vi "subImage.vi"() -> ()   [LabVIEW 2018]
doc: "Sublmage: This example is an example of a sub image, which can be a partial image extracted or captured from the original image."
uses:
  vi.lib/VIRobotics/opencv_yiku/ctls/Point.ctl
  vi.lib/VIRobotics/opencv_yiku/ctls/Rect.ctl
  vi.lib/VIRobotics/opencv_yiku/ctls/ColorConversionCodes.ctl
  vi.lib/VIRobotics/opencv_yiku/Mat/Mat_8U/Mat_8U.lvclass
  D:/Program Files/company/National Instruments/LabVIEW 2018/vi.lib/addons/VIRobotics/opencv_yiku/Mat/Mat/Mat.lvclass
  vi.lib/VIRobotics/opencv_yiku/Mat/Create_Mat_8U.vi
  vi.lib/VIRobotics/opencv_yiku/Cap/Cap.lvclass
  vi.lib/VIRobotics/opencv_yiku/opencv_yiku.lvlib
  vi.lib/VIRobotics/opencv_yiku/Mat/Mat/Mat.lvclass
panel:
  out "sub picture":picture
  out "replace picture":picture
  in  "sub Rect":T1={"x"=100, "y"=100, "width"=200, "height"=100}
  in  "replace start Point":T2={"x"=50, "y"=50}
  out "src picture":picture
  in  "stop":bool
  # "Overview: Demonstrates how to get a subimage and replaceSubImage\nRequirements: Windows.\nInstructions: \n1.Run the VI.\n2.Please note that the selected sub area you set must not exceed the boundaries of the image itself. The area you replace must also not exceed the boundaries of the image itself.\n3.Make sure your computer has a camera."
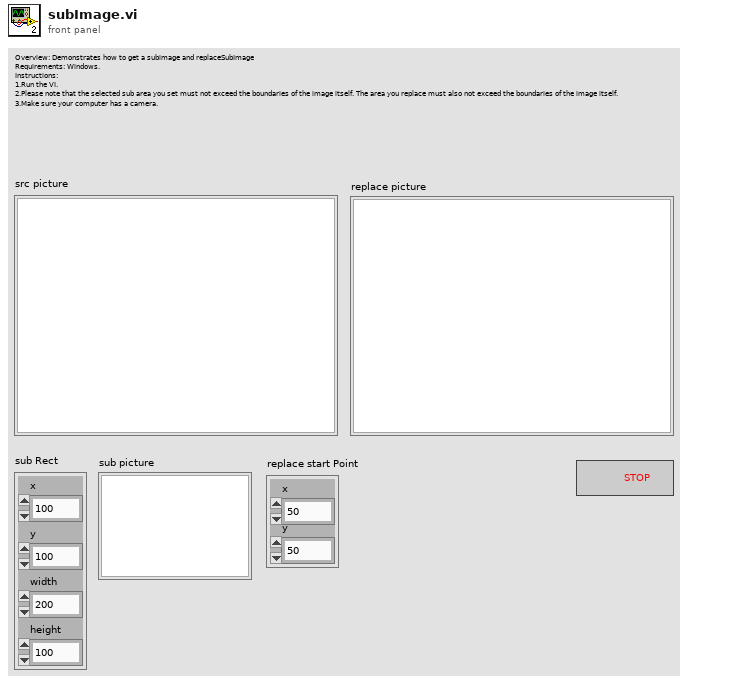
[diagram p1: front panel]
types:
  T1 = typedef "opencv_yiku.lvlib/Rect.ctl" = cluster{"x":i32, "y":i32, "width":i32, "height":i32}
  T2 = typedef "opencv_yiku.lvlib/Point.ctl" = cluster{"x":i32, "y":i32}
  T3 = typedef "opencv_yiku.lvlib/ColorConversionCodes.ctl" = enum32{"COLOR_BGR2BGRA", "COLOR_BGRA2BGR", "COLOR_BGR2RGBA", "COLOR_RGBA2BGR", "COLOR_BGR2RGB", "COLOR_BGRA2RGBA", "COLOR_BGR2GRAY", "COLOR_RGB2GRAY", "COLOR_GRAY2BGR", "COLOR_GRAY2BGRA", "COLOR_BGRA2GRAY", "COLOR_RGBA2GRAY", "COLOR_BGR2BGR565", "COLOR_RGB2BGR565", "COLOR_BGR5652BGR", "COLOR_BGR5652RGB", "COLOR_BGRA2BGR565", "COLOR_RGBA2BGR565", "COLOR_BGR5652BGRA", "COLOR_BGR5652RGBA", "COLOR_GRAY2BGR565", "COLOR_BGR5652GRAY", "COLOR_BGR2BGR555", "COLOR_RGB2BGR555", "COLOR_BGR5552BGR", "COLOR_BGR5552RGB", "COLOR_BGRA2BGR555", "COLOR_RGBA2BGR555", "COLOR_BGR5552BGRA", "COLOR_BGR5552RGBA", "COLOR_GRAY2BGR555", "COLOR_BGR5552GRAY", "COLOR_BGR2XYZ", "COLOR_RGB2XYZ", "COLOR_XYZ2BGR", "COLOR_XYZ2RGB", "COLOR_BGR2YCrCb", "COLOR_RGB2YCrCb", "COLOR_YCrCb2BGR", "COLOR_YCrCb2RGB", "COLOR_BGR2HSV", "COLOR_RGB2HSV", "42", "43", "COLOR_BGR2Lab", "COLOR_RGB2Lab"}
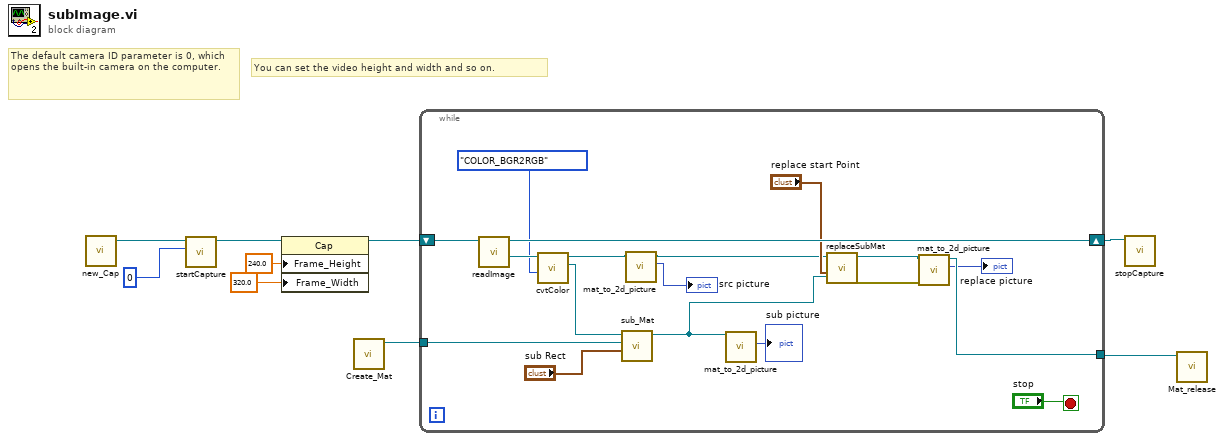
[diagram p0: block diagram]
diagram:
  # "You can set the video height and width and so on."
  # "The default camera ID parameter is 0, which opens the built-in camera on the computer."
  n1 = call "new_Cap.vi"() -> ("Cap out"=w9:refnum<class "Cap.lvclass">)  [unwired: 10 in, 1 out]
  n2 = call "startCapture.vi"("cameraID"=0, "Cap in"=w9) -> ("Cap out"=w6:refnum<class "Cap.lvclass">)  [unwired: 8 in, 1 out]
  n3 = property class="Cap"(reference=w6, "Frame_Height"=240.0, "Frame_Width"=320.0) -> (reference out=w5:refnum<class "Cap.lvclass">)  [unwired: 1 in, 1 out]
  n4 = call-poly "Create_Mat.vi"() -> ("Mat_8U_out"=w3:refnum<class "Mat_8U.lvclass">)  [unwired: 10 in, 1 out]
  n5 = while {
    shift-right: [w26] -> w7
    shift-left: w5 -> [w27]
    tunnel: w3 -> [w23]
    tunnel: [w14] -> w4
    stop <- "stop" stop-if-true
    n6 = call "readImage.vi"("Cap in"=w27) -> ("Mat out"=w24:refnum<class "Mat_8U.lvclass">, "Cap out"=w26:refnum<class "Cap.lvclass">)  [unwired: 8 in, 1 out]
    n7 = call "cvtColor.vi"("dstCn"=ColorConversionCodes."COLOR_BGR2RGB", "src"=w24) -> ("dst out"=w21:refnum<class "Mat_8U.lvclass">, "src out"=w19:refnum<class "Mat_8U.lvclass">)  [unwired: 7 in, 1 out]
    n8 = call "sub_Mat.vi"("Rect"="sub Rect", "dst"=w23, "Mat in"=w21) -> ("dst"=w11:refnum<class "Mat_8U.lvclass">)  [unwired: 7 in, 1 out]
    n9 = call "mat_to_2d_picture.vi"("Mat_8U in"=w19) -> ("picture"=→"src picture":picture, "Mat_8U out"=w18:refnum<class "Mat_8U.lvclass">)  [unwired: 8 in, 1 out]
    n10 = call "mat_to_2d_picture.vi"("Mat_8U in"=w11) -> ("picture"=→"sub picture":picture)  [unwired: 8 in, 2 out]
    n11 = call "replaceSubMat.vi"("SubMat"=w11, "Point"="replace start Point", "src in"=w18) -> ("error out"=w13:errorcluster, "dst out"=w15:refnum<class "Mat_8U.lvclass">)  [unwired: 7 in]
    n12 = call "mat_to_2d_picture.vi"("error in (no error)"=w13, "Mat_8U in"=w15) -> ("picture"=→"replace picture":picture, "Mat_8U out"=w14:refnum<class "Mat_8U.lvclass">)  [unwired: 7 in, 1 out]
  }
  n13 = call "stopCapture.vi"("Cap in"=w7) -> ()  [unwired: 10 in, 1 out]
  n14 = call "Mat_release.vi"("Mat in"=w4) -> ()  [unwired: 10 in, 1 out]
